vi "BuildLabDeltaGraph.vi"(1 "L*a*b intermediary":dbl[][](array[numeric]), 2 "L*a*b 2":dbl[](array[numeric]), 3 "L*a*b 1":dbl[](array[numeric])) -> (0 "L*a*b* Graphs":T1)   [LabVIEW 2013]
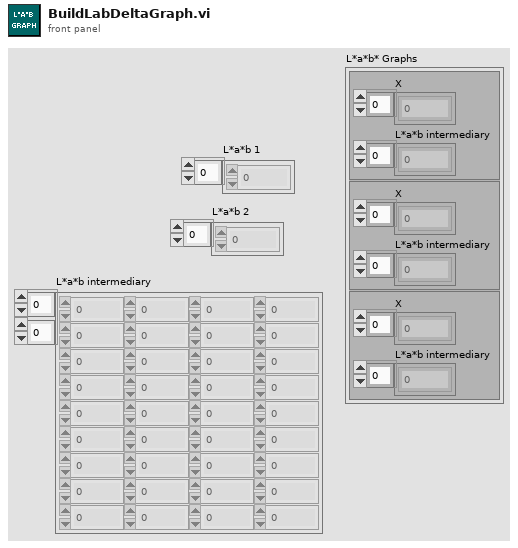
[diagram p1: front panel]
types:
  T1 = cluster{cluster{"X":dbl[], "L*a*b intermediary":dbl[]}, cluster{"X":dbl[], "L*a*b intermediary":dbl[]}, cluster{"X":dbl[], "L*a*b intermediary":dbl[]}}
  T2 = cluster{cluster{i32[], "L*a*b intermediary":dbl[]}, cluster{i32[], "L*a*b intermediary":dbl[]}, cluster{i32[], "L*a*b intermediary":dbl[]}}
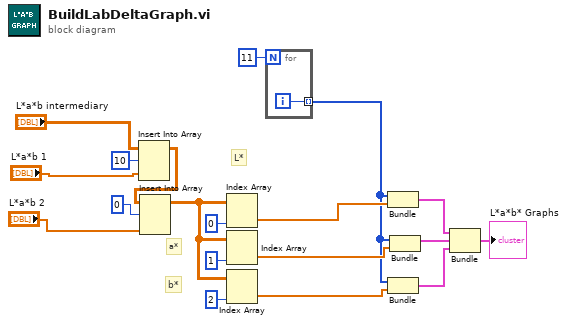
[diagram p0: block diagram]
diagram:
  # "b*"
  # "a*"
  # "L*"
  n1 = Insert Into Array(array="L*a*b intermediary", index (row)=10, new element="L*a*b 1") -> (w16:dbl[][])  [unwired: 1 in]
  n2 = Insert Into Array(array=w16, index (row)=0, new element="L*a*b 2") -> (w10:dbl[][])  [unwired: 1 in]
  n3 = Index Array(array=w10, index (col)=0 ("disabled index (col)")) -> (element=w9:dbl[])  [unwired: 1 in]
  n4 = Index Array(array=w10, index (col)=1 ("disabled index (col)")) -> (element=w8:dbl[])  [unwired: 1 in]
  n5 = Index Array(array=w10, index (col)=2 ("disabled index (col)")) -> (element=w7:dbl[])  [unwired: 1 in]
  n6 = for {
    N: 11 -> [_]
    tunnel: [w20] -> w1 mode=indexing
    i -> [w20]
  }
  n7 = Bundle(w1, "L*a*b intermediary"=w9) -> (w6:cluster{i32[], "L*a*b intermediary":dbl[]})  [unwired: 1 in]
  n8 = Bundle(w1, "L*a*b intermediary"=w7) -> (w4:cluster{i32[], "L*a*b intermediary":dbl[]})  [unwired: 1 in]
  n9 = Bundle(w1, "L*a*b intermediary"=w8) -> (w5:cluster{i32[], "L*a*b intermediary":dbl[]})  [unwired: 1 in]
  n10 = Bundle(w6, w5, w4) -> (→"L*a*b* Graphs":T2)  [unwired: 1 in]
